vi "think_and_act.vi"(8 "error in (no error)":errorcluster, 9 "antState":T1, 10 "pieceOfWorld":T4[][](array[typedef]), 11 "Igor in":refnum<class "Igor.lvclass">) -> (0 "error out":errorcluster, 2 "action":T2, 3 "Igor out":refnum<class "Igor.lvclass">)   [LabVIEW 2015, in "Igor.lvclass"]
doc: "Ant thinks and chooses action\nCreated by Artem Shevelev\nshevelev.pro\nartem@shevelev.pro\nLabVIEW Portal: https://labviewportal.org/memberlist.php?mode=viewprofile&u=2340"
uses:
  Igor.lvclass
  actors/world/typedefs/worldCell_cluster.ctl
  actors/world/typedefs/markValue_cluster.ctl
  actors/world/typedefs/markValue.ctl
  actors/world/typedefs/markVolume.ctl
  actors/world/typedefs/amountOfFood.ctl
  actors/world/typedefs/anthillType_enum.ctl
  ant_base/action_cluster.ctl
  ant_base/actionType_enum.ctl
  ant_base/antState_cluster.ctl
  ant_base/ant_base.lvclass/ant_base.ctl
  ant_base/memory_limit_const.vi
  moving/move_forvard.vi
  moving/move_back.vi
  ant_base/ant_base.lvclass
  actors/world/world.lvlib
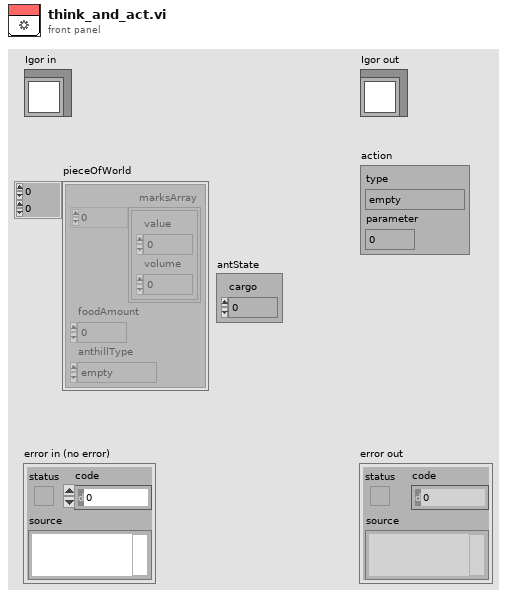
[diagram p1: front panel]
types:
  T1 = typedef "ant_base.lvclass/antState_cluster.ctl" = cluster{"cargo":u8}
  T2 = typedef "ant_base.lvclass/action_cluster.ctl" = cluster{"type":T3, "parameter":dbl}
  T3 = typedef "ant_base.lvclass/actionType_enum.ctl" = enum8{"empty", "move", "take", "put", "mark"}
  T4 = typedef "world.lvlib/worldCell_cluster.ctl" = cluster{"marksArray":T5[], "foodAmount":T8, "anthillType":T9}
  T5 = typedef "world.lvlib/markValue_cluster.ctl" = cluster{"value":T6, "volume":T7}
  T6 = typedef "world.lvlib/markValue.ctl" = u8
  T7 = typedef "world.lvlib/markVolume.ctl" = u16
  T8 = typedef "world.lvlib/amountOfFood.ctl" = i32
  T9 = typedef "world.lvlib/anthillType_enum.ctl" = enum16{"empty", "own", "rival"}
  T10 = typedef "Memory.ctl" = cluster{"Role":i32, "Azimut":i32, "Block Azimut":i32, "Steps I":u32, "Additional steps":i32, "Steps II":u32, " az of transfer":u32, "Provider az":u32, "number of az":u32, "Mark 253":u32}
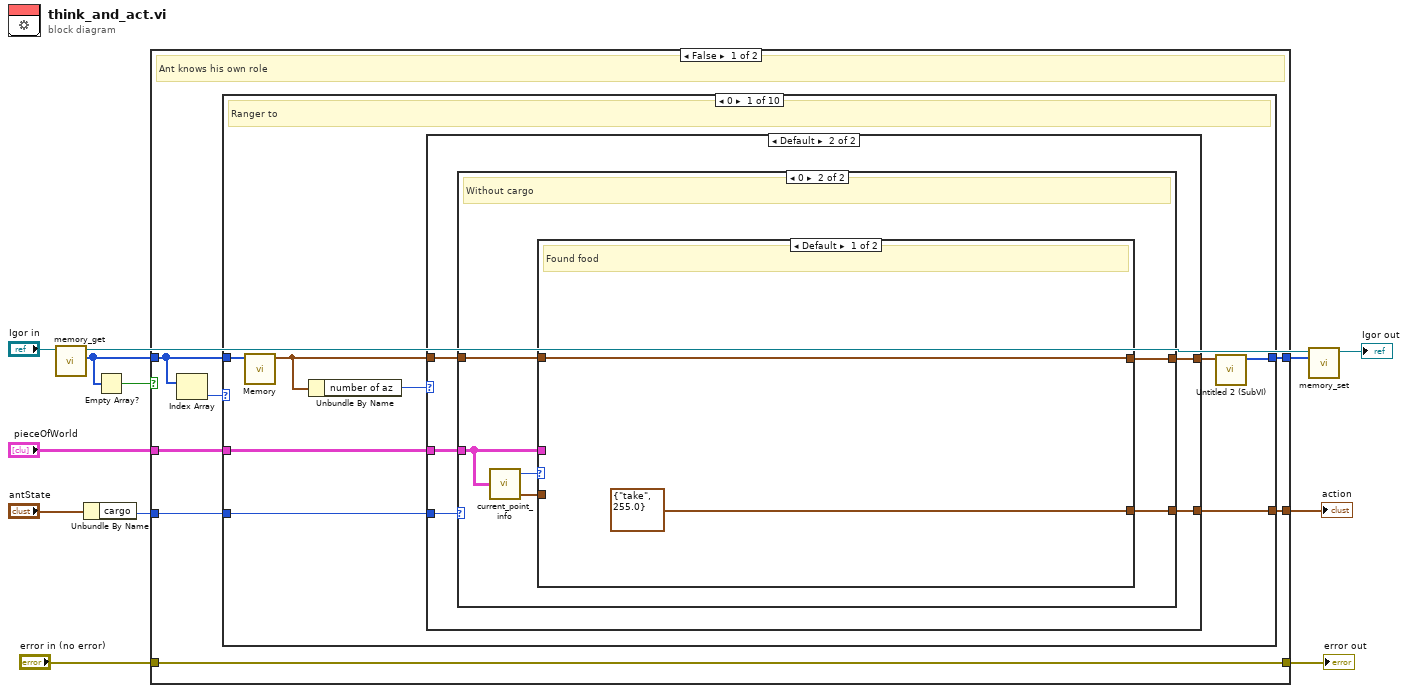
[diagram p0: block diagram]
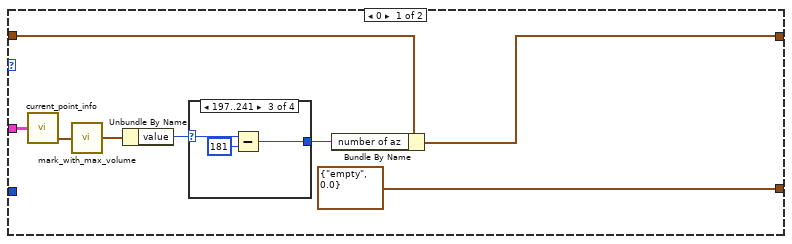
[diagram p2: hidden frame]
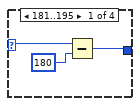
[diagram p3: hidden frame]
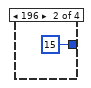
[diagram p4: hidden frame]
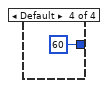
[diagram p5: hidden frame]
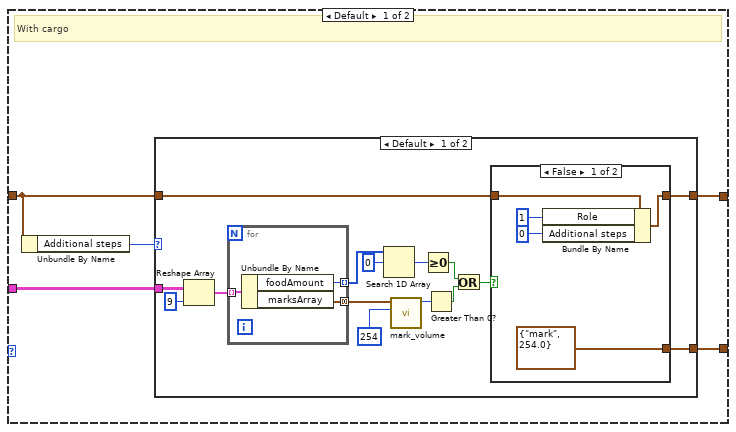
[diagram p6: hidden frame]
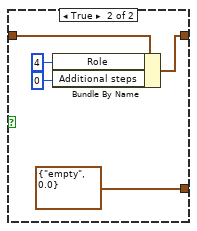
[diagram p7: hidden frame]
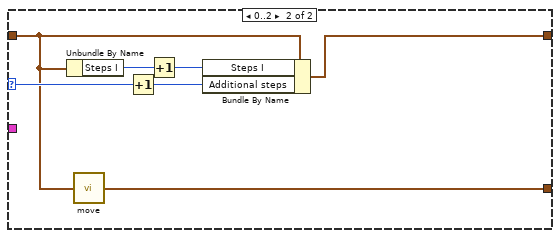
[diagram p8: hidden frame]
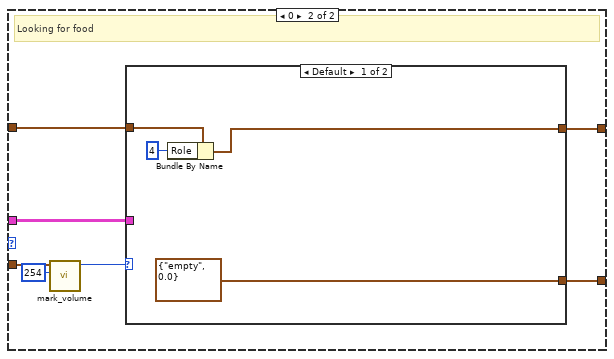
[diagram p9: hidden frame]
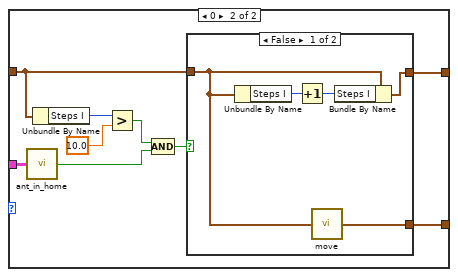
[diagram p10: hidden frame]
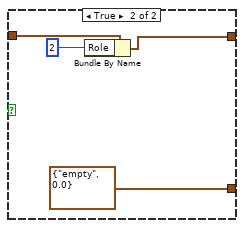
[diagram p11: hidden frame]
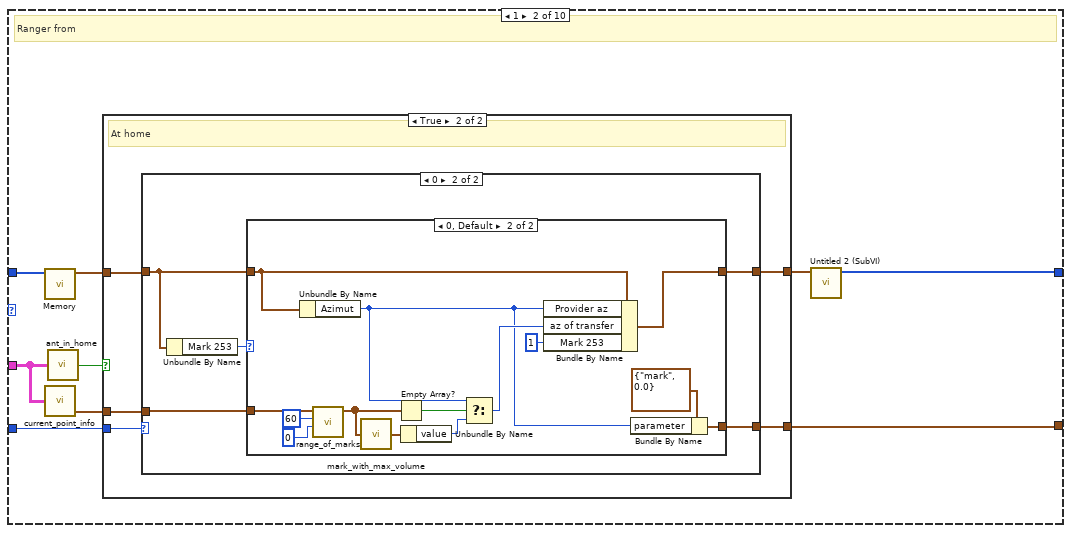
[diagram p12: hidden frame]
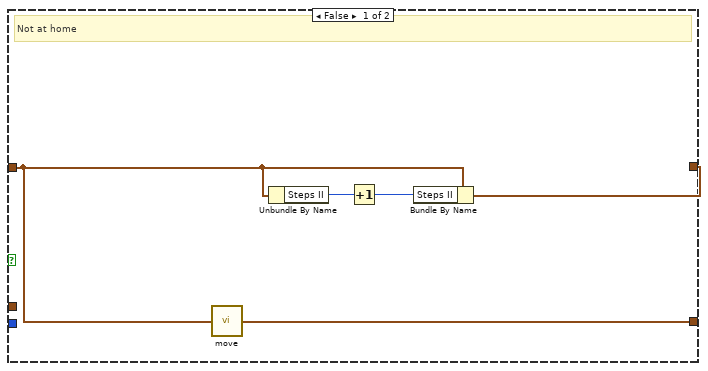
[diagram p13: hidden frame]
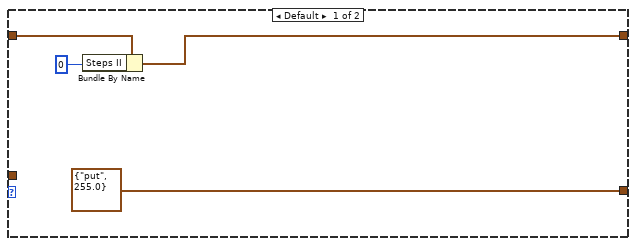
[diagram p14: hidden frame]
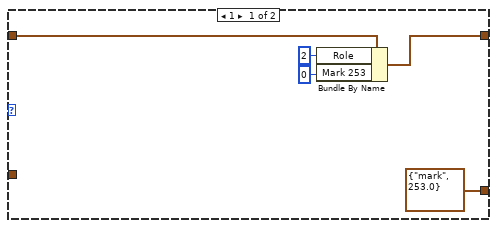
[diagram p15: hidden frame]
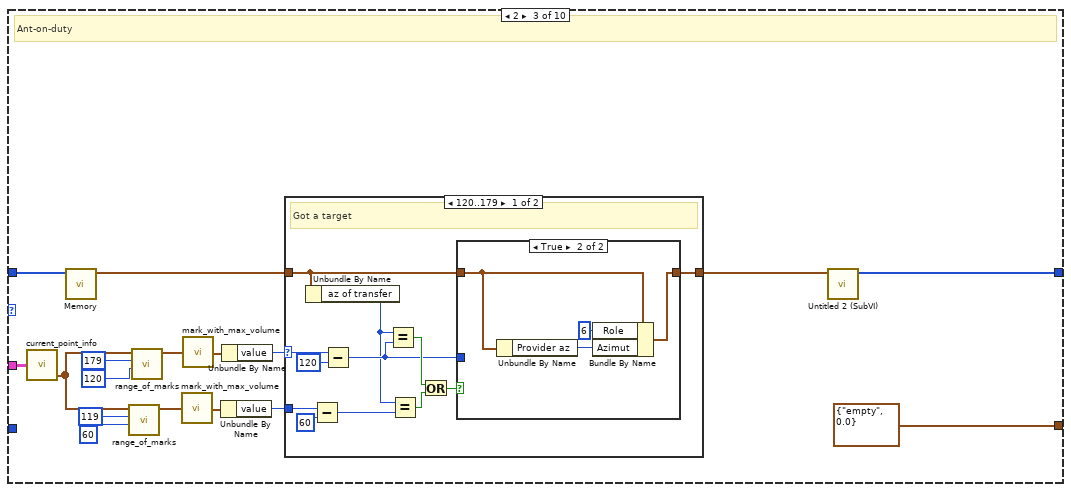
[diagram p16: hidden frame]
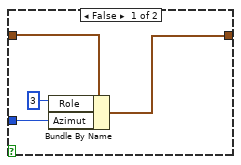
[diagram p17: hidden frame]
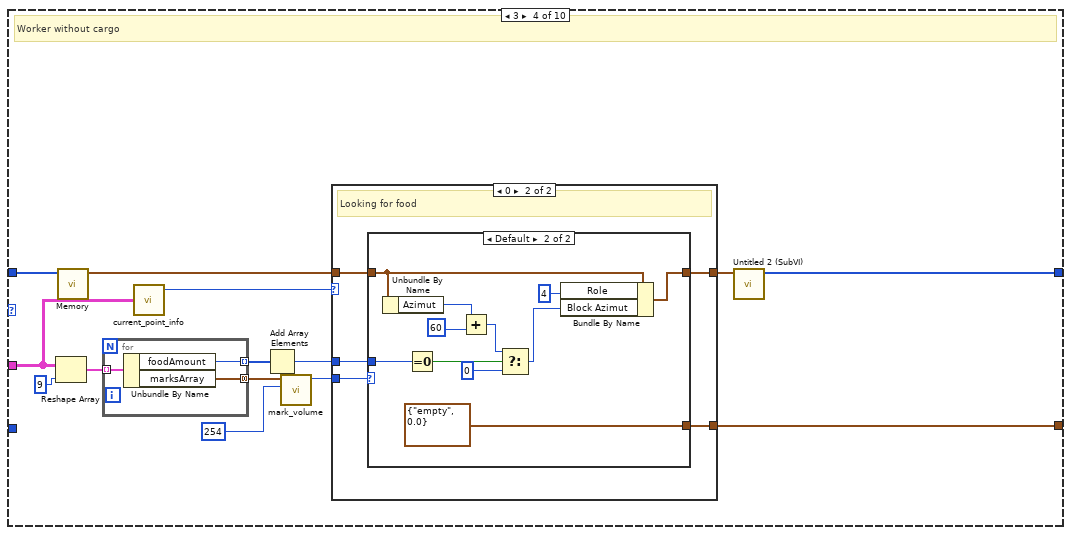
[diagram p19: hidden frame]
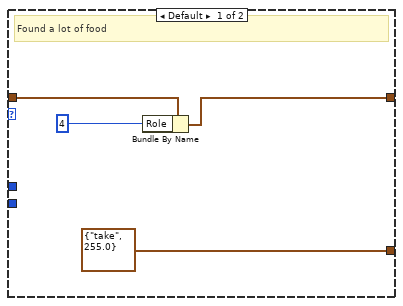
[diagram p20: hidden frame]
diagram:
  n1 = call "memory_get.vi"("ant_base in"="Igor in") -> ("memory"=w2:u8[], "ant_base out"=w7:refnum<class "Igor.lvclass">)  [unwired: 8 in, 1 out]
  n2 = Unbundle By Name("antState") -> ("cargo"=w3:u8)
  n3 = Empty Array?(array=w2) -> (empty?=w9:bool)
  n4 = case shown="False" w9 {
    tunnel: [w19 w620] -> w4
    tunnel: [w17 w619] -> w12
    tunnel: "error in (no error)" -> [w19 w620]
    tunnel: w2 -> [w16 w616]
    tunnel: "pieceOfWorld" -> [w15 w615]
    tunnel: [w14 w617] -> w6
    tunnel: w3 -> [w13 _]
    frame False {
      # "Ant knows his own role"
      n5 = Index Array(array=w16) -> (element=w18:u8)  [unwired: 1 in]
      n6 = case shown="0" w18 {
        tunnel: [w27 w134 T2 {"type"=enum."empty", "parameter"=0.0} ("action") w224 w256 w283 w420 w457 w500 T2 {"type"=enum."empty", "parameter"=0.0} ("action")] -> w17
        tunnel: w16 -> [w24 w129 w176 w214 w253 w282 w418 w453 w496 w612]
        tunnel: w15 -> [w25 w131 w188 w216 w255 w279 w412 w455 w498 _]
        tunnel: [w20 w126 w173 w211 w250 w284 w413 w450 w499 w612] -> w14
        tunnel: w13 -> [w26 w133 _ _ _ _ w422 _ _ _]
        frame 0 {
          # "Ranger to"
          n7 = call "Memory.vi"("memory"=w24) -> ("output cluster"=w22:T10)  [unwired: 10 in]
          n8 = Unbundle By Name(w22) -> ("number of az"=w23:u32)
          n9 = case shown="Default" w23 {
            tunnel: [T2 {"type"=enum."empty", "parameter"=0.0} ("action") w48] -> w27
            tunnel: w22 -> [w28 w47]
            tunnel: [w29 w46] -> w21
            tunnel: w26 -> [_ w45]
            tunnel: w25 -> [w34 w44]
            frame 0 {
              n10 = call "current_point_info.vi"("pieceOfWorld"=w34) -> ("marksArray"=w33:T5[])  [unwired: 2 out]
              n11 = call "mark_with_max_volume.vi"("marksArray"=w33) -> ("markValue"=w32:T5)
              n12 = Unbundle By Name(w32) -> ("value"=w31:T6)
              n13 = case shown="197..241" w31 {
                selector: w31 -> [w38 _ w42 _]
                tunnel: [w36 15 w40 60 ("value")] -> w30
                frame 181..195 {
                  n14 = Subtract(x=w38, y=180 ("index")) -> (x-y=w36:i32)
                }
                frame 196 {
                }
                frame 197..241 {
                  n15 = Subtract(x=w42, y=T6 181) -> (x-y=w40:T6)
                }
                frame Default {
                }
              }
              n16 = Bundle By Name(cluster=w28, "number of az"=w30) -> (w29:T10)
            }
            frame Default {
              n17 = case shown="0" w45 {
                tunnel: [w52 w94] -> w48
                tunnel: w47 -> [w50 w93]
                tunnel: [w53 w92] -> w46
                tunnel: w44 -> [w51 w91]
                frame Default {
                  # "With cargo"
                  n18 = Unbundle By Name(w50) -> ("Additional steps"=w49:i32)
                  n19 = case shown="Default" w49 {
                    selector: w49 -> [_ w88]
                    tunnel: [w66 w85] -> w53
                    tunnel: w50 -> [w67 w84]
                    tunnel: [w68 w87] -> w52
                    tunnel: w51 -> [w65 _]
                    frame Default {
                      n20 = Reshape Array(w65, 9 ("dimension size")) -> (w64:T4[])
                      n21 = for {
                        tunnel: w64 -> [w81] mode=indexing
                        tunnel: [w80] -> w62 mode=concatenating
                        tunnel: [w79] -> w60 mode=indexing
                        n22 = Unbundle By Name(w81) -> ("foodAmount"=w79:T8, "marksArray"=w80:T5[])
                      }
                      n23 = Search 1D Array(1D array=w60, element=T8 0) -> (index of element=w58:i32)  [unwired: 1 in]
                      n24 = call "mark_volume.vi"("element"=T6 254, "marksArray"=w62) -> ("volume"=w57:T7)  [unwired: 9 in]
                      n25 = Greater Or Equal To 0?(x=w58) -> (x >= 0?=w55:bool)
                      n26 = Greater Than 0?(x=w57) -> (x > 0?=w56:bool)
                      n27 = Or(x=w55, y=w56) -> (x .or. y?=w54:bool)
                      n28 = case shown="False" w54 {
                        tunnel: [T2 {"type"=enum."mark", "parameter"=254.0} ("action") T2 {"type"=enum."empty", "parameter"=0.0} ("action")] -> w68
                        tunnel: w67 -> [w71 w76]
                        tunnel: [w72 w77] -> w66
                        frame False {
                          n29 = Bundle By Name(cluster=w71, "Role"=u8 1 ("new element/subarray"), "Additional steps"=u8 0 ("new element/subarray")) -> (w72:T10)
                        }
                        frame True {
                          n30 = Bundle By Name(cluster=w76, "Role"=u8 4 ("new element/subarray"), "Additional steps"=u8 0 ("new element/subarray")) -> (w77:T10)
                        }
                      }
                    }
                    frame 0..2 {
                      n31 = Unbundle By Name(w84) -> ("Steps I"=w86:u32)
                      n32 = call-poly "move.vi"("output cluster"=w84) -> ("action"=w87:T2)
                      n33 = Increment(x=w88) -> (x+1=w82:i32)
                      n34 = Increment(x=w86) -> (x+1=w83:u32)
                      n35 = Bundle By Name(cluster=w84, "Steps I"=w83, "Additional steps"=w82) -> (w85:T10)
                    }
                  }
                }
                frame 0 {
                  # "Without cargo"
                  n36 = call "current_point_info.vi"("pieceOfWorld"=w91) -> ("foodAmount"=w90:T8, "marksArray"=w89:T5[])  [unwired: 1 out]
                  n37 = case shown="Default" w90 {
                    tunnel: [T2 {"type"=enum."take", "parameter"=255.0} ("action") w103] -> w94
                    tunnel: w93 -> [w95 w101]
                    tunnel: [w95 w102] -> w92
                    tunnel: w91 -> [_ w100]
                    tunnel: w89 -> [_ w99]
                    frame Default {
                      # "Found food"
                    }
                    frame 0 {
                      # "Looking for food"
                      n38 = call "mark_volume.vi"("element"=T6 254, "marksArray"=w99) -> ("volume"=w97:T7)  [unwired: 9 in]
                      n39 = case shown="Default" w97 {
                        tunnel: [T2 {"type"=enum."empty", "parameter"=0.0} ("action") w116] -> w103
                        tunnel: [w104 w115] -> w102
                        tunnel: w101 -> [w106 w109]
                        tunnel: w100 -> [_ w111]
                        frame Default {
                          n40 = Bundle By Name(cluster=w106, "Role"=4) -> (w104:T10)
                        }
                        frame 0 {
                          n41 = call "ant_in_home.vi"("pieceOfWorld"=w111) -> ("x .and. y?"=w110:bool)
                          n42 = Unbundle By Name(w109) -> ("Steps I"=w108:u32)
                          n43 = Greater?(x=w108, y=10.0) -> (0:w113:bool)
                          n44 = Compound Arithmetic op=AND(w113, w110) -> (w112:bool)
                          n45 = case shown="False" w112 {
                            tunnel: [w121 T2 {"type"=enum."empty", "parameter"=0.0} ("action")] -> w116
                            tunnel: [w118 w122] -> w115
                            tunnel: w109 -> [w117 w124]
                            frame False {
                              n46 = Unbundle By Name(w117) -> ("Steps I"=w120:u32)
                              n47 = Increment(x=w120) -> (x+1=w119:u32)
                              n48 = call-poly "move.vi"("output cluster"=w117) -> ("action"=w121:T2)
                              n49 = Bundle By Name(cluster=w117, "Steps I"=w119) -> (w118:T10)
                            }
                            frame True {
                              n50 = Bundle By Name(cluster=w124, "Role"=u8 2 ("new element/subarray")) -> (w122:T10)
                            }
                          }
                        }
                      }
                    }
                  }
                }
              }
            }
          }
          n51 = call "Untitled 2 (SubVI).vi"("Cluster"=w21) -> ("appended array"=w20:u32[])  [unwired: 10 in]
        }
        frame 1 {
          # "Ranger from"
          n52 = call "Memory.vi"("memory"=w129) -> ("output cluster"=w128:T10)  [unwired: 10 in]
          n53 = call "current_point_info.vi"("pieceOfWorld"=w131) -> ("marksArray"=w130:T5[])  [unwired: 2 out]
          n54 = call "ant_in_home.vi"("pieceOfWorld"=w131) -> ("x .and. y?"=w132:bool)
          n55 = case shown="True" w132 {
            tunnel: [w139 w144] -> w134
            tunnel: w130 -> [_ w142]
            tunnel: w128 -> [w138 w141]
            tunnel: [w135 w143] -> w127
            tunnel: w133 -> [_ w140]
            frame False {
              # "Not at home"
              n56 = call-poly "move.vi"("output cluster"=w138) -> ("action"=w139:T2)
              n57 = Unbundle By Name(w138) -> ("Steps II"=w137:u32)
              n58 = Increment(x=w137) -> (x+1=w136:u32)
              n59 = Bundle By Name(cluster=w138, "Steps II"=w136) -> (w135:T10)
            }
            frame True {
              # "At home"
              n60 = case shown="0" w140 {
                tunnel: [T2 {"type"=enum."put", "parameter"=255.0} ("action") w151] -> w144
                tunnel: w141 -> [w147 w150]
                tunnel: [w145 w152] -> w143
                tunnel: w142 -> [_ w153]
                frame Default {
                  n61 = Bundle By Name(cluster=w147, "Steps II"=u32 0) -> (w145:T10)
                }
                frame 0 {
                  n62 = Unbundle By Name(w150) -> ("Mark 253"=w149:u32)
                  n63 = case shown="0, Default" w149 {
                    tunnel: w153 -> [_ w172]
                    tunnel: [w154 w159] -> w152
                    tunnel: [T2 {"type"=enum."mark", "parameter"=253.0} ("action") w162] -> w151
                    tunnel: w150 -> [w156 w163]
                    frame 1 {
                      n64 = Bundle By Name(cluster=w156, "Role"=2, "Mark 253"=u32 0) -> (w154:T10)
                    }
                    frame 0, Default {
                      n65 = Unbundle By Name(w163) -> ("Azimut"=w160:i32)
                      n66 = call "range_of_marks.vi"("lower limit"=T6 0, "upper limit"=T6 60, "marksArray"=w172) -> ("Array"=w166:T5[])  [unwired: 8 in]
                      n67 = call "mark_with_max_volume.vi"("marksArray"=w166) -> ("markValue"=w171:T5)
                      n68 = Empty Array?(array=w166) -> (empty?=w170:bool)
                      n69 = Unbundle By Name(w171) -> ("value"=w169:T6)
                      n70 = Select(t=w160, s=w170, f=w169) -> (s? t:f=w165:i32)
                      n71 = Bundle By Name(cluster=w163, "Provider az"=w160, "az of transfer"=w165, "Mark 253"=u32 1) -> (w159:T10)
                      n72 = Bundle By Name(cluster=T2 {"type"=enum."mark", "parameter"=0.0} ("action"), "parameter"=w160) -> (w162:T2)
                    }
                  }
                }
              }
            }
          }
          n73 = call "Untitled 2 (SubVI).vi"("Cluster"=w127) -> ("appended array"=w126:u32[])  [unwired: 10 in]
        }
        frame 2 {
          # "Ant-on-duty"
          n74 = call "current_point_info.vi"("pieceOfWorld"=w188) -> ("marksArray"=w180:T5[])  [unwired: 2 out]
          n75 = call "Memory.vi"("memory"=w176) -> ("output cluster"=w175:T10)  [unwired: 10 in]
          n76 = call "range_of_marks.vi"("lower limit"=T6 60, "upper limit"=T6 119, "marksArray"=w180) -> ("Array"=w179:T5[])  [unwired: 8 in]
          n77 = call "range_of_marks.vi"("lower limit"=T6 120, "upper limit"=T6 179, "marksArray"=w180) -> ("Array"=w184:T5[])  [unwired: 8 in]
          n78 = call "mark_with_max_volume.vi"("marksArray"=w179) -> ("markValue"=w181:T5)
          n79 = call "mark_with_max_volume.vi"("marksArray"=w184) -> ("markValue"=w185:T5)
          n80 = Unbundle By Name(w181) -> ("value"=w177:T6)
          n81 = Unbundle By Name(w185) -> ("value"=w178:T6)
          n82 = case shown="120..179" w178 {
            selector: w178 -> [w197 _]
            tunnel: w175 -> [w191 w210]
            tunnel: [w201 w210] -> w174
            tunnel: w177 -> [w193 _]
            frame 120..179 {
              # "Got a target"
              n83 = Unbundle By Name(w191) -> ("az of transfer"=w190:u32)
              n84 = Subtract(x=w193, y=T6 60) -> (x-y=w192:T6)
              n85 = Subtract(x=w197, y=T6 120) -> (x-y=w195:T6)
              n86 = Equal?(x=w190, y=w195) -> (x = y?=w200:bool)
              n87 = Equal?(x=w190, y=w192) -> (x = y?=w198:bool)
              n88 = Or(x=w200, y=w198) -> (x .or. y?=w199:bool)
              n89 = case shown="True" w199 {
                tunnel: w195 -> [w204 _]
                tunnel: w191 -> [w205 w208]
                tunnel: [w202 w206] -> w201
                frame False {
                  n90 = Bundle By Name(cluster=w205, "Role"=3, "Azimut"=w204) -> (w202:T10)
                }
                frame True {
                  n91 = Unbundle By Name(w208) -> ("Provider az"=w207:u32)
                  n92 = Bundle By Name(cluster=w208, "Role"=6, "Azimut"=w207) -> (w206:T10)
                }
              }
            }
            frame Default {
              # "Expecting a target"
            }
          }
          n93 = call "Untitled 2 (SubVI).vi"("Cluster"=w174) -> ("appended array"=w173:u32[])  [unwired: 10 in]
        }
        frame 3 {
          # "Worker without cargo"
          n94 = Reshape Array(w216, 9 ("dimension size")) -> (w221:T4[])
          n95 = call "Memory.vi"("memory"=w214) -> ("output cluster"=w213:T10)  [unwired: 10 in]
          n96 = for {
            tunnel: w221 -> [w227] mode=indexing
            tunnel: [w226] -> w218 mode=concatenating
            tunnel: [w225] -> w220 mode=indexing
            n97 = Unbundle By Name(w227) -> ("foodAmount"=w225:T8, "marksArray"=w226:T5[])
          }
          n98 = call "current_point_info.vi"("pieceOfWorld"=w216) -> ("foodAmount"=w215:T8)  [unwired: 2 out]
          n99 = Add Array Elements(numeric array=w220) -> (sum=w219:T8)
          n100 = call "mark_volume.vi"("element"=T6 254, "marksArray"=w218) -> ("volume"=w217:T7)  [unwired: 9 in]
          n101 = case shown="0" w215 {
            tunnel: [T2 {"type"=enum."take", "parameter"=255.0} ("action") w236] -> w224
            tunnel: w213 -> [w230 w234]
            tunnel: w217 -> [_ w235]
            tunnel: [w228 w233] -> w212
            tunnel: w219 -> [_ w232]
            frame Default {
              # "Found a lot of food"
              n102 = Bundle By Name(cluster=w230, "Role"=4 ("index")) -> (w228:T10)
            }
            frame 0 {
              # "Looking for food"
              n103 = case shown="Default" w235 {
                tunnel: [w237 T2 {"type"=enum."empty", "parameter"=0.0} ("action")] -> w236
                tunnel: w234 -> [w238 w242]
                tunnel: [w238 w239] -> w233
                tunnel: w232 -> [_ w247]
                frame 0 {
                  n104 = call-poly "move.vi"("output cluster"=w238) -> ("action"=w237:T2)
                }
                frame Default {
                  n105 = Unbundle By Name(w242) -> ("Azimut"=w243:i32)
                  n106 = Equal To 0?(x=w247) -> (x = 0?=w246:bool)
                  n107 = Add(x=w243, y=u8 60) -> (x+y=w245:i32)
                  n108 = Select(t=w245, s=w246, f=u8 0) -> (s? t:f=w240:i32)
                  n109 = Bundle By Name(cluster=w242, "Role"=4, "Block Azimut"=w240) -> (w239:T10)
                }
              }
            }
          }
          n110 = call "Untitled 2 (SubVI).vi"("Cluster"=w212) -> ("appended array"=w211:u32[])  [unwired: 10 in]
        }
        frame 4 {
          # "Worker with cargo"
          n111 = call "ant_in_home.vi"("pieceOfWorld"=w255) -> ("x .and. y?"=w254:bool)
          n112 = call "Memory.vi"("memory"=w253) -> ("output cluster"=w252:T10)  [unwired: 10 in]
          n113 = case shown="True" w254 {
            tunnel: [w257 w262] -> w256
            tunnel: w252 -> [w258 w260]
            tunnel: [w258 w261] -> w251
            frame False {
              # "Not at home"
              n114 = call-poly "move.vi"("output cluster"=w258) -> ("action"=w257:T2)
            }
            frame True {
              # "At home"
              n115 = Unbundle By Name(w260) -> ("Block Azimut"=w259:i32)
              n116 = case shown="60..119" w259 {
                selector: w259 -> [w268 _]
                tunnel: [w269 T2 {"type"=enum."put", "parameter"=255.0} ("action")] -> w262
                tunnel: [w270 w271] -> w261
                tunnel: w260 -> [w267 w274]
                frame 60..119 {
                  n117 = Bundle By Name(cluster=w267, "Role"=u8 2 ("y"), "Block Azimut"=u8 0 ("new element/subarray"), "Mark 253"=u8 0 ("new element/subarray")) -> (w263:T10)
                  n118 = call "mark_253.vi"("mark value"=w268, "Memory in 2"=w263, "Memory in"=w267) -> ("action"=w269:T2, "Memory out"=w270:T10)  [unwired: 7 in]
                }
                frame Default {
                  n119 = Bundle By Name(cluster=w274, "Role"=2, "Block Azimut"=0) -> (w271:T10)
                }
              }
            }
          }
          n120 = call "Untitled 2 (SubVI).vi"("Cluster"=w251) -> ("appended array"=w250:u32[])  [unwired: 10 in]
        }
        frame 55 {
          n121 = call "current_point_info.vi"("pieceOfWorld"=w279) -> ("anthillType"=w285:T9)  [unwired: 2 out]
          n122 = Reshape Array(w279, 9 ("dimension size")) -> (w277:T4[])
          n123 = Index Array(array=w282, index=4) -> (element=w280:u8)
          n124 = for {
            tunnel: w277 -> [w287] mode=indexing
            tunnel: [w286] -> w276 mode=concatenating
            n125 = Unbundle By Name(w287) -> ("marksArray"=w286:T5[])
          }
          n126 = case shown="2" w280 {
            tunnel: w285 -> [w291 _ _]
            tunnel: w282 -> [w290 w345 w374]
            tunnel: [w289 w344 w373] -> w284
            tunnel: [w288 w343 w372] -> w283
            tunnel: w276 -> [_ _ w371]
            frame 0, Default {
              n127 = case shown="Default" w291 {
                tunnel: w290 -> [w296 w308]
                tunnel: [w303 w307] -> w289
                tunnel: [w301 w306] -> w288
                frame "own" {
                  n128 = Index Array(array=w296, index=1) -> (element=w298:u8)
                  n129 = Index Array(array=w296, index=2) -> (element=w294:u8)
                  n130 = Increment(x=w294) -> (x+1=w292:u8)
                  n131 = Multiply(x=w298, y=1.5707963267948966) -> (x*y=w297:dbl)
                  n132 = Replace Array Subset(array=w296, new element=w292, index=2) -> (w303:u8[])
                  n133 = Bundle By Name(cluster=T2 {"type"=enum."move", "parameter"=0.0} ("action"), "parameter"=w297) -> (w301:T2)
                }
                frame Default {
                  n134 = Index Array(array=w308, index #1=3 ("index"), index #2=2 ("index")) -> (element #1=w305:u8, element #2=w304:u8)
                  n135 = Greater Or Equal?(x=w305, y=w304) -> (x >= y?=w309:bool)
                  n136 = case shown="False" w309 {
                    tunnel: w308 -> [w315 w329]
                    tunnel: [w322 w335] -> w307
                    tunnel: [w312 T2 {"type"=enum."empty", "parameter"=0.0} ("action")] -> w306
                    tunnel: w305 -> [w320 _]
                    frame False {
                      n137 = Increment(x=w320) -> (x+1=w319:u8)
                      n138 = Index Array(array=w315, index=1) -> (element=w316:u8)
                      n139 = Multiply(x=w316, y=1.5707963267948966) -> (x*y=w314:dbl)
                      n140 = Replace Array Subset(array=w315, new element=w319, index=3) -> (w322:u8[])
                      n141 = Bundle By Name(cluster=T2 {"type"=enum."move", "parameter"=0.0} ("action"), "parameter"=w314) -> (w312:T2)
                    }
                    frame True {
                      n142 = Index Array(array=w329, index=1) -> (element=w327:u8)
                      n143 = Increment(x=w327) -> (x+1=w326:u8)
                      n144 = Quotient & Remainder(x=w326, y=u8 4) -> (x-y*floor(x/y)=w324:u8)  [unwired: 1 out]
                      n145 = Replace Array Subset(array=w329, new element #1=u8 0 ("new element/subarray"), index #1=3 ("index"), new element #2=u8 1 ("new element/subarray"), index #2=4 ("index"), new element #3=w324, index #3=1 ("index")) -> (w335:u8[])
                    }
                  }
                }
              }
            }
            frame 1 {
              n146 = Index Array(array=w345, index #1=3 ("index"), index #2=2 ("index")) -> (element #1=w339:u8, element #2=w337:u8)
              n147 = Multiply(x=w337, y=u8 2) -> (x*y=w336:u8)
              n148 = Greater Or Equal?(x=w339, y=w336) -> (x >= y?=w340:bool)
              n149 = case shown="False" w340 {
                tunnel: w345 -> [w350 w363]
                tunnel: [w346 w369] -> w344
                tunnel: [w347 T2 {"type"=enum."empty", "parameter"=0.0} ("action")] -> w343
                tunnel: w339 -> [w355 _]
                frame False {
                  n150 = Increment(x=w355) -> (x+1=w354:u8)
                  n151 = Replace Array Subset(array=w350, new element=w354, index=3) -> (w346:u8[])
                  n152 = Index Array(array=w346, index=1) -> (element=w351:u8)
                  n153 = Multiply(x=w351, y=1.5707963267948966) -> (x*y=w349:dbl)
                  n154 = Bundle By Name(cluster=T2 {"type"=enum."move", "parameter"=0.0} ("action"), "parameter"=w349) -> (w347:T2)
                }
                frame True {
                  n155 = Index Array(array=w363, index=1) -> (element=w361:u8)
                  n156 = Increment(x=w361) -> (x+1=w360:u8)
                  n157 = Quotient & Remainder(x=w360, y=u8 4) -> (x-y*floor(x/y)=w358:u8)  [unwired: 1 out]
                  n158 = Replace Array Subset(array=w363, new element #1=u8 0 ("new element/subarray"), index #1=3 ("index"), new element #2=u8 2 ("new element/subarray"), index #2=4 ("index"), new element #3=w358, index #3=1 ("index")) -> (w369:u8[])
                }
              }
            }
            frame 2 {
              n159 = Empty Array?(array=w371) -> (empty?=w370:bool)
              n160 = case shown="False" w370 {
                tunnel: w374 -> [w384 w409]
                tunnel: [w383 w409] -> w373
                tunnel: [w382 T2 {"type"=enum."mark", "parameter"=23.0} ("action")] -> w372
                frame False {
                  n161 = Index Array(array=w384, index #1=3 ("index"), index #2=2 ("index")) -> (element #1=w378:u8, element #2=w377:u8)
                  n162 = Multiply(x=w377, y=u8 4) -> (x*y=w375:u8)
                  n163 = Greater Or Equal?(x=w378, y=w375) -> (x >= y?=w379:bool)
                  n164 = case shown="True" w379 {
                    tunnel: w384 -> [w389 w402]
                    tunnel: [w385 w408] -> w383
                    tunnel: [w386 T2 {"type"=enum."empty", "parameter"=0.0} ("action")] -> w382
                    tunnel: w378 -> [w394 _]
                    frame False {
                      n165 = Increment(x=w394) -> (x+1=w393:u8)
                      n166 = Replace Array Subset(array=w389, new element=w393, index=3) -> (w385:u8[])
                      n167 = Index Array(array=w385, index=1) -> (element=w390:u8)
                      n168 = Multiply(x=w390, y=1.5707963267948966) -> (x*y=w388:dbl)
                      n169 = Bundle By Name(cluster=T2 {"type"=enum."move", "parameter"=0.0} ("action"), "parameter"=w388) -> (w386:T2)
                    }
                    frame True {
                      n170 = Index Array(array=w402, index=1) -> (element=w400:u8)
                      n171 = Increment(x=w400) -> (x+1=w399:u8)
                      n172 = Quotient & Remainder(x=w399, y=u8 4) -> (x-y*floor(x/y)=w397:u8)  [unwired: 1 out]
                      n173 = Replace Array Subset(array=w402, new element #1=u8 0 ("new element/subarray"), index #1=3 ("index"), new element #2=u8 2 ("new element/subarray"), index #2=4 ("index"), new element #3=w397, index #3=1 ("index")) -> (w408:u8[])
                    }
                  }
                }
                frame True {
                }
              }
            }
          }
        }
        frame 6 {
          # "Expirienced ranger to foodHeap"
          n174 = call "Memory.vi"("memory"=w418) -> ("output cluster"=w417:T10)  [unwired: 10 in]
          n175 = Unbundle By Name(w417) -> ("Steps II"=w416:u32, "Steps I"=w415:u32)
          n176 = call "current_point_info.vi"("pieceOfWorld"=w412) -> ("foodAmount"=w419:T8)  [unwired: 2 out]
          n177 = call "ant_in_home.vi"("pieceOfWorld"=w412) -> ("x .and. y?"=w411:bool)
          n178 = Greater Or Equal?(x=w416, y=w415) -> (x >= y?=w421:bool)
          n179 = case shown="True" w421 {
            tunnel: w422 -> [w427 w445]
            tunnel: w419 -> [w428 _]
            tunnel: w417 -> [w430 w441]
            tunnel: [w423 T2 {"type"=enum."mark", "parameter"=254.0} ("action")] -> w420
            tunnel: [w429 w438] -> w414
            tunnel: w411 -> [_ _]
            frame False {
              n180 = Greater Than 0?(x=w427) -> (x > 0?=w425:bool)
              n181 = Greater Than 0?(x=w428) -> (x > 0?=w426:bool)
              n182 = Implies(1:w425, 2:w426) -> (0:w424:bool)
              n183 = case shown="True" w424 {
                tunnel: [w431 w433] -> w429
                tunnel: w430 -> [w431 w435]
                tunnel: [T2 {"type"=enum."take", "parameter"=255.0} ("action") w437] -> w423
                frame False {
                  # "Found food"
                }
                frame True {
                  # "No food in cell"
                  n184 = Unbundle By Name(w435) -> ("Steps II"=w436:u32)
                  n185 = call-poly "move.vi"("output cluster"=w435) -> ("action"=w437:T2)
                  n186 = Increment(x=w436) -> (x+1=w434:u32)
                  n187 = Bundle By Name(cluster=w435, "Steps II"=w434) -> (w433:T10)
                }
              }
            }
            frame True {
              n188 = Unbundle By Name(w441) -> ("Azimut"=w442:i32)
              n189 = Less?(x=w445, y=u8 255) -> (x < y?=w443:bool)
              n190 = Add(x=w442, y=u8 60) -> (x+y=w447:i32)
              n191 = Select(t=w447, s=w443, f=u8 0) -> (s? t:f=w439:i32)
              n192 = Bundle By Name(cluster=w441, "Role"=7, "Block Azimut"=w439) -> (w438:T10)
            }
          }
          n193 = call "Untitled 2 (SubVI).vi"("Cluster"=w414) -> ("appended array"=w413:u32[])  [unwired: 10 in]
        }
        frame 7 {
          # "Expirienced ranger from foodHeap"
          n194 = call "Memory.vi"("memory"=w453) -> ("output cluster"=w452:T10)  [unwired: 10 in]
          n195 = call "current_point_info.vi"("pieceOfWorld"=w455) -> ("marksArray"=w454:T5[])  [unwired: 2 out]
          n196 = call "ant_in_home.vi"("pieceOfWorld"=w455) -> ("x .and. y?"=w456:bool)
          n197 = case shown="True" w456 {
            tunnel: [w458 w467] -> w457
            tunnel: w452 -> [w459 w461]
            tunnel: [w459 w466] -> w451
            tunnel: w454 -> [_ w465]
            frame False {
              # "Not at home"
              n198 = call-poly "move.vi"("output cluster"=w459) -> ("action"=w458:T2)
            }
            frame True {
              # "At home"
              n199 = Unbundle By Name(w461) -> ("Azimut"=w460:i32)
              n200 = Add(x=w460, y=u8 60) -> (x+y=w463:i32)
              n201 = call "mark_volume.vi"("element"=w463, "marksArray"=w465) -> ("volume"=w462:T7)  [unwired: 9 in]
              n202 = case shown="Default" w462 {
                tunnel: [T2 {"type"=enum."put", "parameter"=255.0} ("action") w476] -> w467
                tunnel: w461 -> [w470 w474]
                tunnel: [w468 w475] -> w466
                tunnel: w460 -> [_ _]
                frame Default {
                  w469 = 0 ("Block Azimut")
                  n203 = Bundle By Name(cluster=w470, "Role"=2, "Azimut"=w469, "Block Azimut"=w469, "Steps I"=w469, "Additional steps"=w469, "Steps II"=w469, "az of transfer"=w469, "Provider az"=w469, "Mark 253"=w469) -> (w468:T10)
                }
                frame 0 {
                  n204 = Unbundle By Name(w474) -> ("Block Azimut"=w473:i32)
                  n205 = case shown="Default" w473 {
                    selector: w473 -> [_ w489]
                    tunnel: w474 -> [w481 w485]
                    tunnel: [T2 {"type"=enum."put", "parameter"=255.0} ("action") w490] -> w476
                    tunnel: [w477 w491] -> w475
                    frame 0 {
                      n206 = Bundle By Name(cluster=w481, "Role"=6, "Block Azimut"=0, "Steps II"=u32 0) -> (w477:T10)
                    }
                    frame Default {
                      n207 = Bundle By Name(cluster=w485, "Role"=7, "Block Azimut"=0, "Steps II"=u32 0, "Mark 253"=u32 0) -> (w483:T10)
                      n208 = call "mark_253.vi"("mark value"=w489, "Memory in 2"=w483, "Memory in"=w485) -> ("action"=w490:T2, "Memory out"=w491:T10)  [unwired: 7 in]
                    }
                  }
                }
              }
            }
          }
          n209 = call "Untitled 2 (SubVI).vi"("Cluster"=w451) -> ("appended array"=w450:u32[])  [unwired: 10 in]
        }
        frame 180 {
          # "gap"
          # "Administrator"
          n210 = Array Subset(array=w496, index=4, length=3) -> (w493:u8[])
          n211 = call "current_point_info.vi"("pieceOfWorld"=w498) -> ("marksArray"=w497:T5[])  [unwired: 2 out]
          n212 = call "256_to_10.vi"("Array"=w493) -> ("Numeric"=w492:dbl)
          n213 = case shown="Default" w492 {
            selector: w492 -> [_ w518]
            tunnel: [T2 {"type"=enum."empty", "parameter"=0.0} ("action") w530] -> w500
            tunnel: w496 -> [w505 w519]
            tunnel: [w508 w529] -> w499
            tunnel: w497 -> [w510 w528]
            frame 0 {
              n214 = call "mark_with_max_volume.vi"("marksArray"=w510) -> ("markValue"=w509:T5)
              n215 = Unbundle By Name(w509) -> ("volume"=w507:T7)
              n216 = Array Subset(array=w505, index=1, length=3) -> (w502:u8[])
              n217 = call "256_to_10.vi"("Array"=w502) -> ("Numeric"=w501:dbl)
              n218 = Subtract(x=w501, y=w507) -> (x-y=w506:dbl)
              n219 = case shown="Default" w506 {
                selector: w506 -> [_ w513]
                tunnel: w505 -> [w512 w517]
                tunnel: [w512 w514] -> w508
                frame 0 {
                }
                frame Default {
                  n220 = call "10_to_256.vi"("Decimal"=w513) -> ("256"=w515:u8[])
                  n221 = Replace Array Subset(array=w517, new element=w515, index=4) -> (w514:u8[])
                }
              }
            }
            frame Default {
              # "max"
              n222 = Array Subset(array=w519, index=1, length=3) -> (w522:u8[])
              n223 = call "mark_volume.vi"("element"=T6 253, "marksArray"=w528) -> ("volume"=w521:T7)  [unwired: 9 in]
              n224 = call "256_to_10.vi"("Array"=w522) -> ("Numeric"=w520:dbl)
              n225 = Subtract(x=w520, y=w521) -> (x-y=w526:dbl)
              n226 = Less Or Equal?(x=w526, y=w518) -> (x <= y?=w525:bool)
              n227 = case shown="True" w525 {
                tunnel: [w537 T2 {"type"=enum."empty", "parameter"=0.0} ("action")] -> w530
                tunnel: w519 -> [w533 w565]
                tunnel: [w533 w559] -> w529
                tunnel: w528 -> [w535 w569]
                tunnel: w521 -> [_ w567]
                tunnel: w518 -> [_ w566]
                frame False {
                  n228 = Array Subset(array=w533, index=7) -> (w531:u8[])  [unwired: 1 in]
                  n229 = call "mark_volume.vi"("element"=T6 180, "marksArray"=w535) -> ("volume"=w536:T7)  [unwired: 9 in]
                  n230 = case shown="Default" w536 {
                    tunnel: [w540 T2 {"type"=enum."mark", "parameter"=180.0} ("action")] -> w537
                    tunnel: w531 -> [w538 _]
                    tunnel: w535 -> [w539 _]
                    frame Default {
                      n231 = for {
                        tunnel: [w544] -> w540
                        tunnel: w539 -> [w543]
                        tunnel: w538 -> [w541] mode=indexing
                        stop <- w542 stop-if-true
                        n232 = case shown="0..59" w541 {
                          selector: w541 -> [_ w547]
                          tunnel: [T2 {"type"=enum."empty", "parameter"=0.0} ("action") w553] -> w544
                          tunnel: w543 -> [_ w552]
                          tunnel: [FALSE TRUE] -> w542
                          frame Default {
                          }
                          frame 0..59 {
                            n233 = Add(x=w547, y=u8 120) -> (x+y=w550:u8)
                            n234 = call "mark_volume.vi"("element"=w550, "marksArray"=w552) -> ("volume"=w549:T7)  [unwired: 9 in]
                            n235 = case shown="0..1000" w549 {
                              tunnel: [T2 {"type"=enum."empty", "parameter"=0.0} ("action") w557] -> w553
                              tunnel: w550 -> [_ w556]
                              frame Default {
                              }
                              frame 0..1000 {
                                n236 = Bundle By Name(cluster=T2 {"type"=enum."mark", "parameter"=0.0} ("action"), "parameter"=w556) -> (w557:T2)
                              }
                            }
                          }
                        }
                      }
                    }
                    frame 0..1000 {
                    }
                  }
                }
                frame True {
                  n237 = Delete From Array(array=w565, length=7, index=0) -> (deleted portion=w561:u8[], array with subset deleted=w562:u8[])
                  n238 = for {
                    tunnel: w569 -> [w578] mode=indexing
                    shift-right: [w576] -> w560
                    shift-left: w562 -> [w577]
                    tunnel: w567 -> [w571]
                    tunnel: w566 -> [w572]
                    n239 = Unbundle By Name(w578) -> ("volume"=w570:T7, "value"=w575:T6)
                    n240 = Subtract(x=w571, y=w570) -> (x-y=w574:T7)
                    n241 = Less Or Equal?(x=w574, y=w572) -> (x <= y?=w573:bool)
                    n242 = case shown="True" w573 {
                      tunnel: w577 -> [w579 w582]
                      tunnel: [w579 w581] -> w576
                      tunnel: w575 -> [_ w580]
                      frame False {
                      }
                      frame True {
                        n243 = case shown="0..59" w580 {
                          selector: w580 -> [_ w588 w601]
                          tunnel: w582 -> [w583 w589 w603]
                          tunnel: [w583 w586 w602] -> w581
                          frame Default {
                          }
                          frame 0..59 {
                            n244 = Add(x=w588, y=T6 60) -> (x+y=w591:T6)
                            n245 = Search 1D Array(1D array=w589, element=w588) -> (index of element=w584:i32)  [unwired: 1 in]
                            n246 = Search 1D Array(1D array=w589, element=w591) -> (index of element=w585:i32)  [unwired: 1 in]
                            n247 = case shown="-1" w584 {
                              tunnel: w589 -> [w596 w599]
                              tunnel: [w596 w598] -> w587
                              tunnel: w588 -> [_ w597]
                              frame Default {
                              }
                              frame -1 {
                                n248 = Insert Into Array(array=w599, new element=w597) -> (w598:u8[])  [unwired: 1 in]
                              }
                            }
                            n249 = case shown="Default" w585 {
                              selector: w585 -> [_ w593]
                              tunnel: w587 -> [w592 w595]
                              tunnel: [w592 w594] -> w586
                              frame -1 {
                              }
                              frame Default {
                                n250 = Delete From Array(array=w595, index=w593) -> (array with subset deleted=w594:u8[])  [unwired: 1 in, 1 out]
                              }
                            }
                          }
                          frame 60..119 {
                            n251 = Search 1D Array(1D array=w603, element=w601) -> (index of element=w600:i32)  [unwired: 1 in]
                            n252 = case shown="-1" w600 {
                              tunnel: w603 -> [w604 w609]
                              tunnel: [w604 w607] -> w602
                              tunnel: w601 -> [_ w606]
                              frame 0, Default {
                              }
                              frame -1 {
                                n253 = Subtract(x=w606, y=T6 60) -> (x-y=w611:T6)
                                n254 = Insert Into Array(array=w609, new element=w606) -> (w608:u8[])  [unwired: 1 in]
                                n255 = Search 1D Array(1D array=w609, element=w611) -> (index of element=w605:i32)  [unwired: 1 in]
                                n256 = Delete From Array(array=w608, index=w605) -> (array with subset deleted=w607:u8[])  [unwired: 1 in, 1 out]
                              }
                            }
                          }
                        }
                      }
                    }
                  }
                  n257 = Insert Into Array(array=w561, new element=w560) -> (w559:u8[])  [unwired: 1 in]
                }
              }
            }
          }
        }
        frame Default {
        }
      }
    }
    frame True {
      # "Ant's memory is empty"
      n258 = call "current_point_info.vi"("pieceOfWorld"=w615) -> ("marksArray"=w614:T5[])  [unwired: 2 out]
      n259 = Empty Array?(array=w614) -> (empty?=w618:bool)
      n260 = case shown="False" w618 {
        tunnel: [w626 w675] -> w619
        tunnel: [w625 w671] -> w617
        tunnel: w616 -> [_ _]
        tunnel: w614 -> [w624 _]
        frame False {
          n261 = call "mark_with_max_volume.vi"("marksArray"=w624) -> ("markValue"=w623:T5)
          n262 = Unbundle By Name(w623) -> ("volume"=w621:T7, "value"=w622:T6)
          n263 = case shown="181..194" w622 {
            selector: w622 -> [w633 w641 w649 w657 w665]
            tunnel: [w631 w645 w653 w661 w668] -> w626
            tunnel: [w637 w644 w652 w660 w666] -> w625
            tunnel: w621 -> [w632 _ _ _ _]
            frame 180 {
              w627 = T6 0 ("element")
              n264 = call "10_to_256.vi"("Decimal"=w632) -> ("256"=w636:u8[])
              n265 = Index Array(array=w636) -> (element #1=w629:u8, element #2=w630:u8, element #3=w628:u8)  [unwired: 3 in]
              n266 = Build Array(T6 180 ("element"), w629, w630, w628, w627, w627, w627) -> (w637:T6[])
              n267 = Increment(x=w633) -> (x+1=w634:T6)
              n268 = Bundle By Name(cluster=T2 {"type"=enum."mark", "parameter"=0.0} ("action"), "parameter"=w634) -> (w631:T2)
            }
            frame 181..194 {
              w639 = T6 0 ("element")
              # "Ant became a ranger"
              n269 = Increment(x=w641) -> (x+1=w643:T6)
              n270 = Subtract(x=w641, y=T6 180) -> (x-y=w640:T6)
              n271 = Build Array(w639, w640, w639, w639, w639, w639, w639, w639, w639, w639, w639, w639, w639, w639) -> (w644:T6[])
              n272 = Bundle By Name(cluster=T2 {"type"=enum."mark", "parameter"=0.0} ("action"), "parameter"=w643) -> (w645:T2)
            }
            frame 195 {
              w647 = T6 0 ("y")
              # "Ant became a ranger"
              n273 = Increment(x=w649) -> (x+1=w650:T6)
              n274 = Build Array(T6 5 ("element"), T6 0 ("element"), w647, w647, w647, w647, w647, w647, w647, w647, w647, w647, w647, w647) -> (w652:T6[])
              n275 = Bundle By Name(cluster=T2 {"type"=enum."mark", "parameter"=0.0} ("action"), "parameter"=w650) -> (w653:T2)
            }
            frame 196..240 {
              w655 = T6 0 ("element")
              # "Ant became a ranger"
              n276 = Increment(x=w657) -> (x+1=w659:T6)
              n277 = Subtract(x=w657, y=T6 181) -> (x-y=w656:T6)
              n278 = Build Array(w655, w656, w655, w655, w655, w655, w655, w655, w655, w655, w655, w655, w655, w655) -> (w660:T6[])
              n279 = Bundle By Name(cluster=T2 {"type"=enum."mark", "parameter"=0.0} ("action"), "parameter"=w659) -> (w661:T2)
            }
            frame Default {
              w663 = T6 0 ("element")
              # "Ant became an ant-on-duty"
              n280 = Build Array(T6 2 ("element"), w663, w663, w663, w663, w663, w663, w663, w663, w663, w663, w663, T6 60 ("element"), w663) -> (w666:T6[])
              n281 = Bundle By Name(cluster=T2 {"type"=enum."mark", "parameter"=0.0} ("action"), "parameter"=w665) -> (w668:T2)
            }
          }
        }
        frame True {
          w670 = T6 0 ("element")
          # "The very first ant"
          n282 = Bundle By Name(cluster=T2 {"type"=enum."mark", "parameter"=0.0} ("action"), "parameter"=T6 180 ("element")) -> (w675:T2)
          n283 = Build Array(w670, T6 0 ("element"), w670, w670, w670, w670, w670, w670, w670, w670, w670, w670, w670, w670) -> (w671:T6[])
        }
      }
    }
  }
  "error out" <- w4
  "action" <- w12
  n284 = call "memory_set.vi"("memory"=w6, "ant_base in"=w7) -> ("ant_base out"=→"Igor out":refnum<class "Igor.lvclass">)  [unwired: 8 in, 1 out]
